vi "Microscope Settings Frame Counter.vi"(1 "Microscope Settings in":T1={"Mode"=enum."Brightfield", "Slit"={"Scanning Mode"=0.0, "Slit Width /%"=0.0}, "Colour"=[], "Exposure/ms"=0.0, "Piezo Position /um"=0.0, "ROI"={"X"={"Start /px"=0.0, "Step /px"=0.0, "Range /px"=0.0}, "Y"={"Start /px"=0.0, "Step /px"=0.0, "Range /px"=0.0}, "Z "={"Start /um"=0.0, "Step/um"=0.0, "Range /um"=0.0}, "T "={"Start /s"=0.0, "Step /s"=0.0, "Range /s"=0.0}}, "Samples per millisecond"=0.0, "Relax/ms"=0.0, "Readout Direction"=0.0, "Trigger Source"=0.0, "Camera Delay /ms"=0.0, "Under Scan /ms"=0.0, "Waveforms"={"Analogue Out"=[], "Digital Out"=[]}, "Slit Scanning Delay /ms"=11.0} {"Slit Scanning Delay /ms" min=0.0 max=10.0 step=0.05; "Under Scan /ms" min=0.0 max=10.0 step=0.05; "ROI"."T"."Range /s" min=0.0 max=10.0 step=0.05; "ROI"."T"."Step /s" min=0.0 max=10.0 step=0.05; "ROI"."T"."Start /s" min=0.0 max=10.0 step=0.05; "ROI"."X"."Range /px" min=0.0 max=10.0 step=0.05; "ROI"."X"."Step /px" min=0.0 max=10.0 step=0.05; "ROI"."X"."Start /px" min=0.0 max=10.0 step=0.05; "ROI"."Y"."Range /px" min=0.0 max=10.0 step=0.05; "ROI"."Y"."Step /px" min=0.0 max=10.0 step=0.05; "ROI"."Y"."Start /px" min=0.0 max=10.0 step=0.05; "ROI"."Z"."Range /um" min=0.0 max=10.0 step=0.05; "ROI"."Z"."Step/um" min=0.0 max=10.0 step=0.05; "ROI"."Z"."Start /um" min=0.0 max=10.0 step=0.05; "Colour"."Colour"."Filter" items=["Empty"=1, ""=2, ""=3, "561"=4, ""=5, "488"=6]; "Camera Delay /ms" min=0.0 max=10.0 step=0.05; "Trigger Source" items=["Internal"=1.0, "External"=2.0]; "Readout Direction" items=["Forward"=1.0, "Backward"=2.0]; "Slit"."Scanning Mode" items=["Full Frame"=1.0, "Slit Scanning"=12.0]; "Piezo Position /um" min=0.0 max=10.0 step=0.05}) -> (0 "Frames":i32)   [LabVIEW 2016]
uses:
  controls/Microscope Settings.ctl
  controls/ColourCalibration.ctl
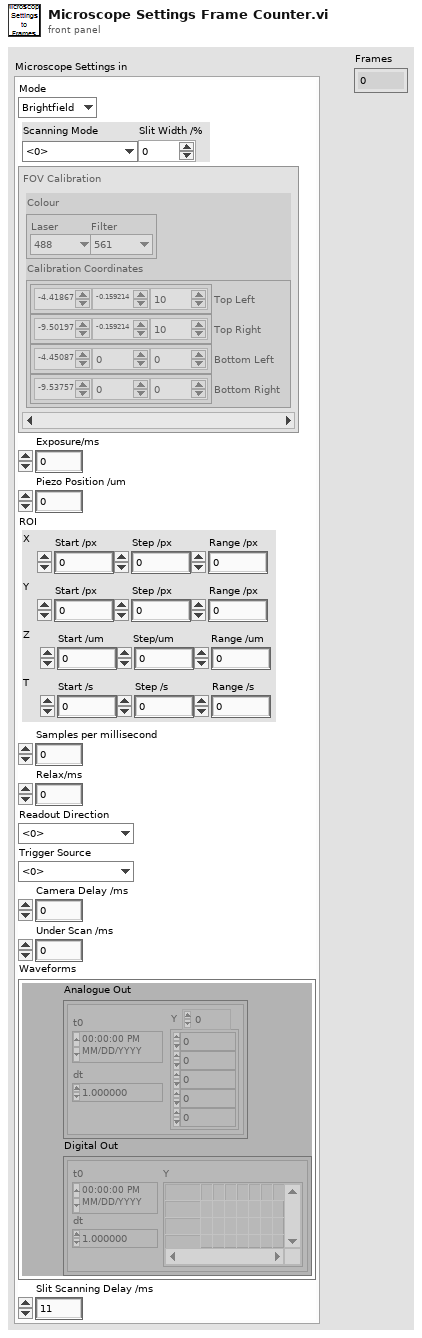
[diagram p1: front panel]
types:
  T1 = typedef "Microscope Settings.ctl" = cluster{"Mode":enum16{"Brightfield", "X", "XY", "XYZ", "XYZT", "XYZC", "Tweezers", "Virus"}, "Slit":cluster{"Scanning Mode":dbl, "Slit Width /%":dbl}, "Colour":T2, "Exposure/ms":dbl, "Piezo Position /um":dbl, "ROI":cluster{"X":cluster{"Start /px":dbl, "Step /px":dbl, "Range /px":dbl}, "Y":cluster{"Start /px":dbl, "Step /px":dbl, "Range /px":dbl}, "Z ":cluster{"Start /um":dbl, "Step/um":dbl, "Range /um":dbl}, "T ":cluster{"Start /s":dbl, "Step /s":dbl, "Range /s":dbl}}, "Samples per millisecond":dbl, "Relax/ms":dbl, "Readout Direction":dbl, "Trigger Source":dbl, "Camera Delay /ms":dbl, "Under Scan /ms":dbl, "Waveforms":cluster{"Analogue Out":waveform(dbl)[], "Digital Out":digitalwaveform[]}, "Slit Scanning Delay /ms":dbl}
  T2 = typedef "ColourCalibration.ctl" = cluster{"Colour":cluster{"Laser":enum16{"Brightfield", "445", "488", "561", "647"}, "Filter":u16}, "Calibration Coordinates":cluster{"Top Left":dbl[], "Top Right":dbl[], "Bottom Left":dbl[], "Bottom Right":dbl[]}}[]
  T3 = enum16{"Brightfield", "X", "XY", "XYZ", "XYZT", "XYZC", "Tweezers", "Virus"}
  T4 = cluster{"Start /um":dbl, "Step/um":dbl, "Range /um":dbl}
  T5 = cluster{"Start /s":dbl, "Step /s":dbl, "Range /s":dbl}
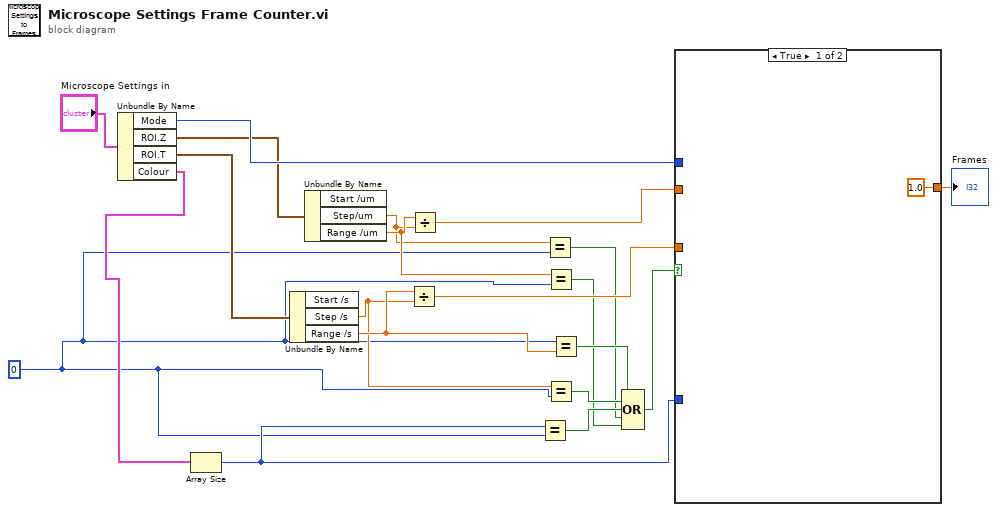
[diagram p0: block diagram]
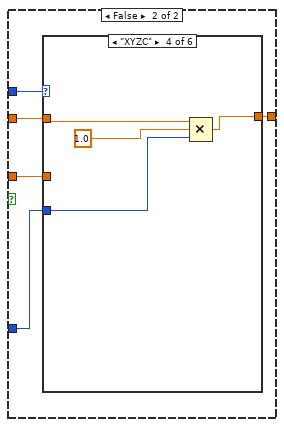
[diagram p2: hidden frame]
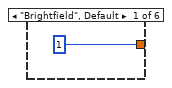
[diagram p3: hidden frame]
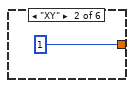
[diagram p4: hidden frame]
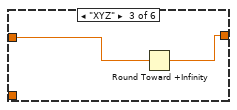
[diagram p5: hidden frame]
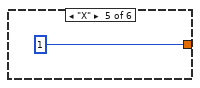
[diagram p6: hidden frame]
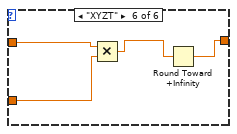
[diagram p7: hidden frame]
diagram:
  w4 = 0 ("y")
  n1 = Unbundle By Name("Microscope Settings in") -> ("Mode"=w19:T3, "ROI.Z"=w17:T4, "ROI.T"=w16:T5, "Colour"=w13:T2)
  n2 = Array Size(array=w13) -> (size(s)=w12:i32)
  n3 = Unbundle By Name(w16) -> ("Step /s"=w10:dbl, "Range /s"=w11:dbl)  [unwired: 1 out]
  n4 = Unbundle By Name(w17) -> ("Step/um"=w5:dbl, "Range /um"=w6:dbl)  [unwired: 1 out]
  n5 = Divide(x=w11, y=w10) -> (x/y=w14:dbl)
  n6 = Divide(x=w6, y=w5) -> (x/y=w15:dbl)
  n7 = Equal?(x=w12, y=w4) -> (x = y?=w9:bool)
  n8 = Equal?(x=w5, y=w4) -> (x = y?=w3:bool)
  n9 = Equal?(x=w6, y=w4) -> (x = y?=w2:bool)
  n10 = Equal?(x=w10, y=w4) -> (x = y?=w8:bool)
  n11 = Equal?(x=w4, y=w11) -> (x = y?=w7:bool)
  n12 = Compound Arithmetic op=OR(w7, w8, w9, w3, w2) -> (w1:bool)
  n13 = case shown="True" w1 {
    tunnel: w19 -> [_ w26]
    tunnel: [1.0 ("Frames") w25] -> w18
    tunnel: w15 -> [_ w24]
    tunnel: w14 -> [_ w23]
    tunnel: w12 -> [_ w22]
    frame True {
    }
    frame False {
      n14 = case shown="\"XYZC\"" w26 {
        tunnel: [1 ("Frames") 1 ("Frames") w29 w33 1 ("Frames") w36] -> w25
        tunnel: w24 -> [_ _ w30 w34 _ w39]
        tunnel: w23 -> [_ _ _ _ _ w38]
        tunnel: w22 -> [_ _ _ w32 _ _]
        frame "Brightfield", Default {
        }
        frame "XY" {
        }
        frame "XYZ" {
          n15 = Round Toward +Infinity(x=w30) -> (ceil(x): smallest int >= x=w29:dbl)
        }
        frame "XYZC" {
          n16 = Compound Arithmetic op=MULTIPLY(w34, 1.0 ("value"), w32) -> (w33:dbl)
        }
        frame "X" {
        }
        frame "XYZT" {
          n17 = Multiply(x=w39, y=w38) -> (x*y=w37:dbl)
          n18 = Round Toward +Infinity(x=w37) -> (ceil(x): smallest int >= x=w36:dbl)
        }
      }
    }
  }
  "Frames" <- w18
